vi "Flip (Greyscale Y-Axis).vi"(8 "error in (no error)":errorcluster, 10 "Greyscale Destination Image in":T1, 11 "Greyscale Source Image in":T1) -> (0 "error out":errorcluster, 3 "Greyscale Destination Image":T1)   [LabVIEW 2020, in "image.lvlib"]
doc: "Flip the image around the Y axis."
uses:
  image.lvlib
  Greyscale Image.ctl
  Flip Mode.ctl
  348de330-10c9-445f-8d54-7780e9118077.vi
  <vilib>/Utility/error.llb/Error Cluster From Error Code.vi
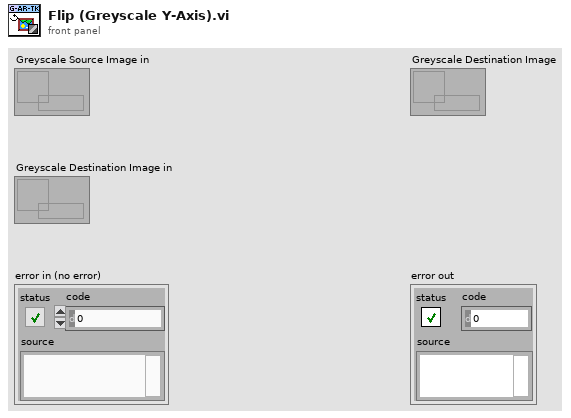
[diagram p1: front panel]
types:
  T1 = typedef "image.lvlib/Greyscale Image.ctl" = refnum<data-value>
  T2 = typedef "image.lvlib/Flip Mode.ctl" = enum8{"X-Axis", "Y-Axis", "X and Y Axes"}
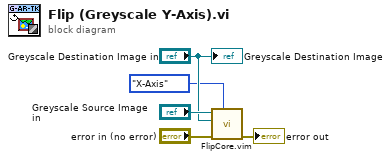
[diagram p0: block diagram]
diagram:
  n1 = call "FlipCore.vim"("Flip Mode"=Flip_Mode."X-Axis" ("Flip Mode (Default: X-Axis)"), "error in (no error)"="error in (no error)", "Destination Image"="Greyscale Destination Image in", "Source Image"="Greyscale Source Image in") -> ("error out"=→"error out":errorcluster)  [unwired: 7 in]
  "Greyscale Destination Image" <- "Greyscale Destination Image in"
